vi "Process DAQ Data.vi"(0 "reset averaging":bool, 1 "Processing loop variables":T6 {"CurrInverter"."last updated" format="%<%H:%M\n%d/%m/%Y>T"; "CurrInverter"."set flag" items=["False", "True"]}, 2 "Data Rate 9775(S/s)":dbl=3.0 format="%#.6p", 3 "RawDAQData in":T16, 4 "Signal scaling":T15[](array[typedef]), 5 "error in":errorcluster, 6 "Data Rate 9215 (S/s)":dbl=1200000.0 format="%#.6p", 7 "ESR scaling":T14[](array[typedef]), 8 "Acquisition mode":T1, 11 "Use dummy Vout?":bool, 13 "Dummy Vrms":dbl=120.0) -> (10 "InverterWaveforms":T2, 15 "Processing loop vars out":T6 {"CurrInverter"."last updated" format="%<%H:%M\n%d/%m/%Y>T"; "CurrInverter"."set flag" items=["False", "True"]}, 16 "DataProcAuxData":T13[](array[typedef]), 18 "MeasData":T4, 19 "error out":errorcluster)   [LabVIEW 2019, in "Main.lvclass"]
doc: "Developed by Kevin Thompson\nkevin@thompsonengineering.net\n\nCopyright 2020\nThompson Engineering, LLC"
uses:
  Main.lvclass
  Common/DataTypes/RawDAQData--cluster.ctl
  Common/DataTypes/RawChannelData--cluster.ctl
  subvis/DataTypes/Gain control.ctl
  subvis/DataTypes/Processing loop variables--cluster.ctl
  subvis/DataTypes/averaging variables.ctl
  subvis/DataTypes/ESR alarm variables.ctl
  Common/DataTypes/Inverter database record v2--cluster.ctl
  Common/DataTypes/inverter info v2--cluster.ctl
  Common/DataTypes/inverter gain range--cluster.ctl
  Common/DataTypes/inverter offset range--cluster.ctl
  subvis/DataTypes/ESR scaling--cluster.ctl
  DataTypes/DataProcessAuxData--cluster.ctl
  Common/DataQ_SE/TD MeasData--cluster.ctl
  Common/DataTypes/InverterPhaseData--cluster.ctl
  Common/DataTypes/InverterWaveforms--cluster.ctl
  Common/DataTypes/ChannelWaveforms--cluster.ctl
  Common/DataTypes/Acquisition Mode--cluster.ctl
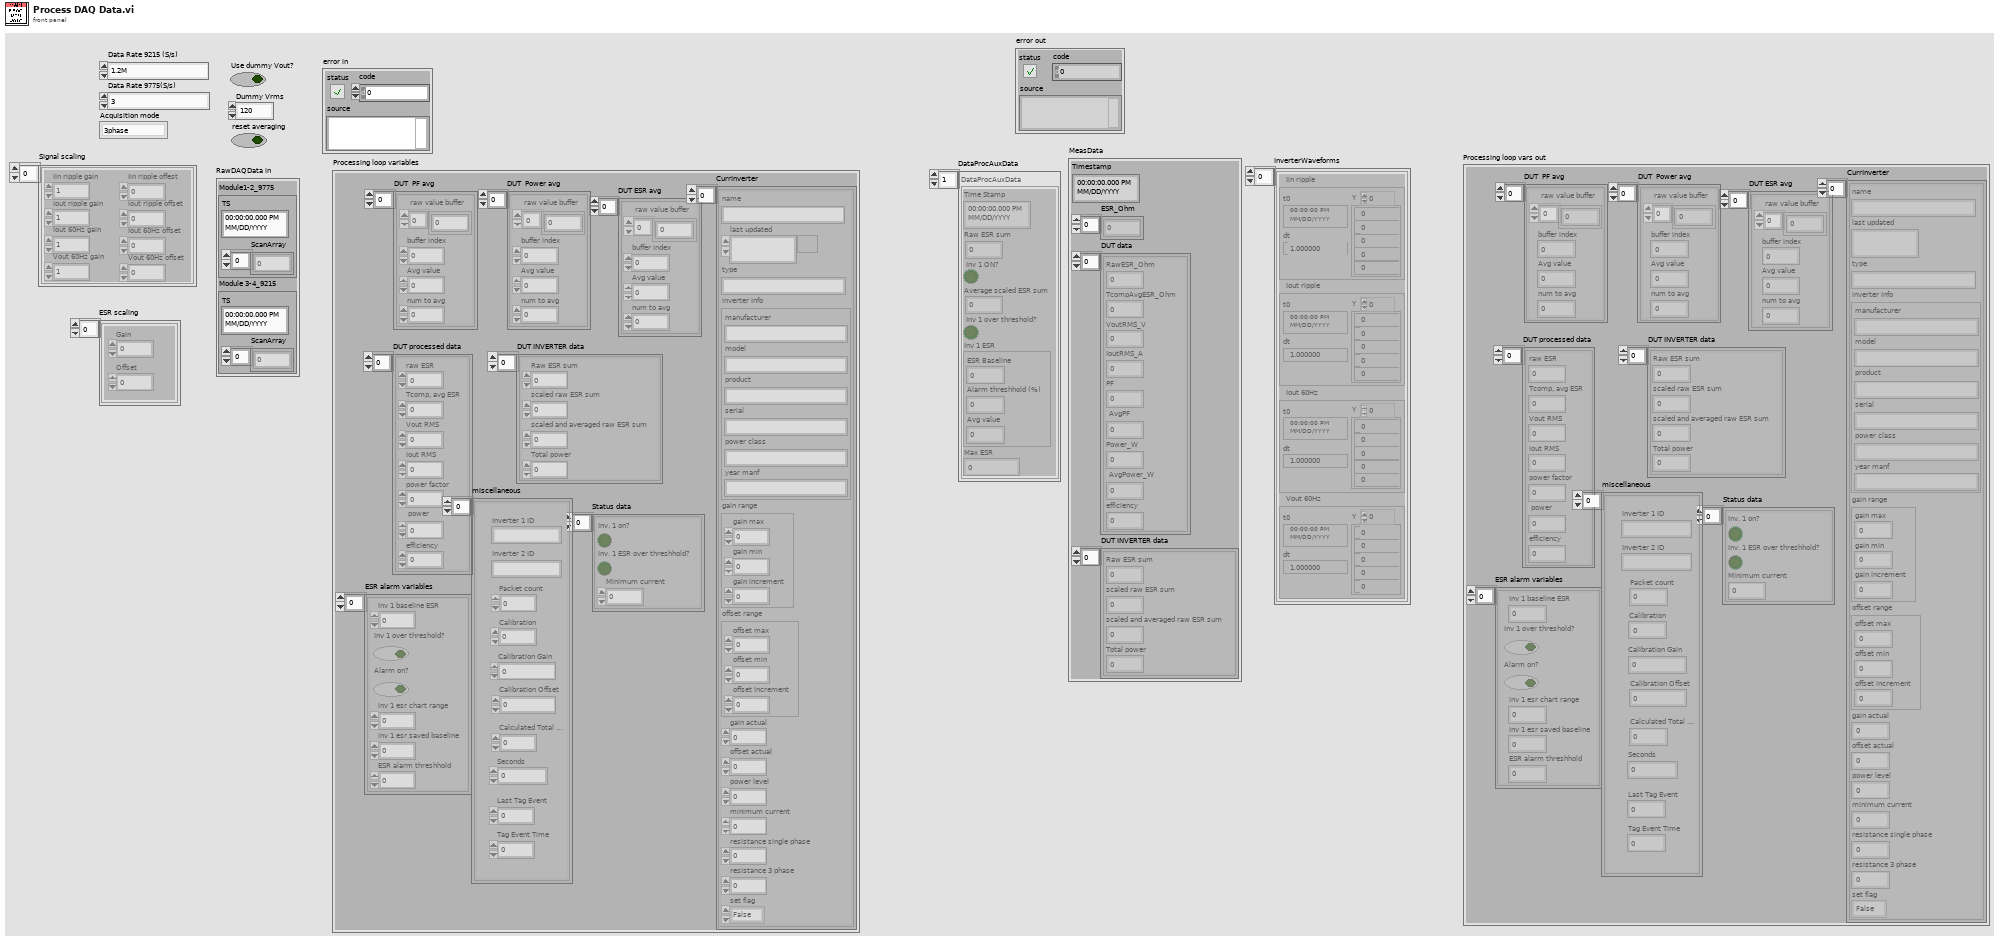
[diagram p1: front panel]
types:
  T1 = typedef "Acquisition Mode--cluster.ctl" = enum16{"3phase", "Single"}
  T2 = typedef "InverterWaveforms--cluster.ctl" = T3[]
  T3 = typedef "ChannelWaveforms--cluster.ctl" = cluster{"Iin ripple ":waveform(dbl), "Iout ripple ":waveform(dbl), "Iout 60Hz":waveform(dbl), "Vout 60Hz":waveform(dbl)}
  T4 = typedef "TD MeasData--cluster.ctl" = cluster{"Timestamp":timestamp, "ESR_Ohm":dbl[], "DUT data":T5[], "DUT INVERTER data":cluster{"Raw ESR sum":dbl, "scaled raw ESR sum":dbl, "scaled and averaged raw ESR sum":dbl, "Total power":dbl}[]}
  T5 = typedef "InverterPhaseData--cluster.ctl" = cluster{"RawESR_Ohm":dbl, "TcompAvgESR_Ohm":dbl, "VoutRMS_V":dbl, "IoutRMS_A":dbl, "PF":dbl, "AvgPF":dbl, "Power_W":dbl, "AvgPower_W":dbl, "efficiency":dbl}
  T6 = typedef "Main.lvclass/Processing loop variables--cluster.ctl" = cluster{"DUT ESR avg":T7[], "DUT  PF avg":T7[], "DUT  Power avg ":T7[], "DUT processed data":cluster{"raw ESR":dbl, "Tcomp, avg ESR":dbl, "Vout RMS":dbl, "Iout RMS":dbl, "power factor":dbl, "power":dbl, "efficiency":dbl}[], "ESR alarm variables":T8[], "Status data":cluster{"Inv. 1 on?":bool, "Inv. 1 ESR over threshhold?":bool, "Minimum current":dbl}[], "CurrInverter":T9[], "miscellaneous":cluster{"Inverter 1 ID":string, "Inverter 2 ID":string, "Packet count":u32, "Calibration":dbl, "Calibration Gain":dbl, "Calibration Offset":dbl, "Calculated Total Power":dbl, "Seconds":dbl, "Last Tag Event":dbl, "Tag Event Time":dbl}[], "DUT INVERTER data":cluster{"Raw ESR sum":dbl, "scaled raw ESR sum":dbl, "scaled and averaged raw ESR sum":dbl, "Total power":dbl}[]}
  T7 = typedef "Main.lvclass/averaging variables.ctl" = cluster{"raw value buffer":dbl[], "buffer index":i32, "Avg value":dbl, "num to avg":i32}
  T8 = typedef "Main.lvclass/ESR alarm variables.ctl" = cluster{"Inv 1 baseline ESR":dbl, "Inv 1 over threshold?":bool, "Alarm on?":bool, "inv 1 esr chart range":dbl, "inv 1 esr saved baseline":dbl, "ESR alarm threshhold":dbl}
  T9 = typedef "Inverter database record v2--cluster.ctl" = cluster{"name":string, "last updated":timestamp, "type":string, "inverter Info":T10, "gain range":T11, "offset range":T12, "gain actual":dbl, "offset actual":dbl, "power level":dbl, "minimum current":dbl, "resistance single phase":dbl, "resistance 3 phase":dbl, "set flag":u16}
  T10 = typedef "inverter info v2--cluster.ctl" = cluster{"manufacturer":string, "model":string, "product":string, "serial":string, "power class":string, "year manf":string}
  T11 = typedef "inverter gain range--cluster.ctl" = cluster{"gain max":dbl, "gain min":dbl, "gain increment":dbl}
  T12 = typedef "inverter offset range--cluster.ctl" = cluster{"offset max":dbl, "offset min":dbl, "offset increment":dbl}
  T13 = typedef "DataProcessAuxData--cluster.ctl" = cluster{"Time Stamp":timestamp, "Raw ESR sum":dbl, "Inv 1 ON?":bool, "Average scaled ESR sum":dbl, "Inv 1 over threshold?":bool, "Inv 1 ESR":cluster{"ESR Baseline":dbl, "Alarm threshhold (%)":dbl, "Avg value":dbl}, "Max ESR":dbl}
  T14 = typedef "Main.lvclass/ESR scaling--cluster.ctl" = cluster{"Gain":dbl, "Offset":dbl}
  T15 = typedef "Main.lvclass/Gain control.ctl" = cluster{"Iin ripple gain":dbl, "Iout ripple gain":dbl, "Iout 60Hz gain ":dbl, "Vout 60Hz gain ":dbl, "Iin ripple offest":dbl, "Iout ripple offset":dbl, "Iout 60Hz offset":dbl, "Vout 60Hz offset":dbl}
  T16 = typedef "RawDAQData--cluster.ctl" = cluster{"Module1-2_9775":T17, "Module 3-4_9215":T17}
  T17 = typedef "RawChannelData--cluster.ctl" = cluster{"TS":timestamp, "ScanArray":dbl[]}
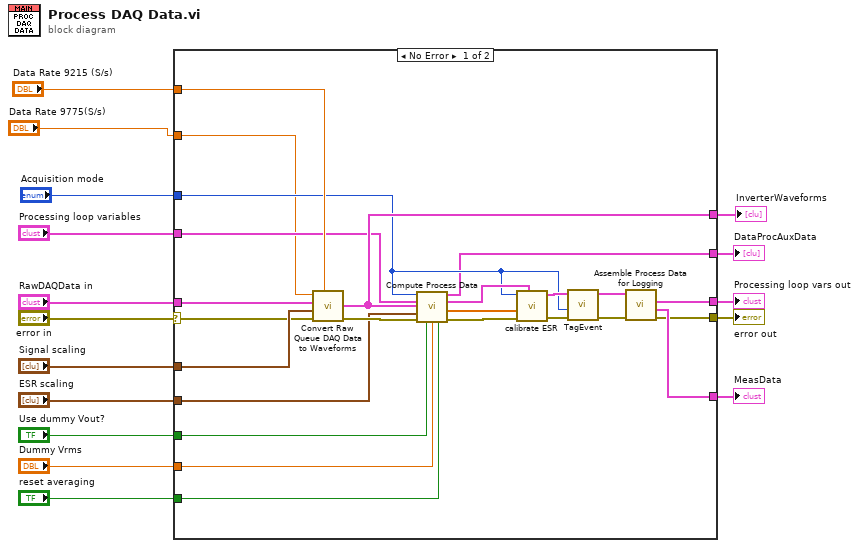
[diagram p0: block diagram]
diagram:
  n1 = case shown="No Error" "error in" {
    selector: "error in" -> [w28 w42]
    tunnel: "RawDAQData in" -> [w39 _]
    tunnel: "Data Rate 9215 (S/s)" -> [w38 _]
    tunnel: "Signal scaling" -> [w37 _]
    tunnel: "Processing loop variables" -> [w27 w41]
    tunnel: "ESR scaling" -> [w36 _]
    tunnel: "Use dummy Vout?" -> [w35 _]
    tunnel: "Dummy Vrms" -> [w34 _]
    tunnel: "reset averaging" -> [w33 _]
    tunnel: [w19 _] -> w8
    tunnel: [w32 w41] -> w7
    tunnel: [w31 _] -> w6
    tunnel: [w30 w42] -> w5
    tunnel: [w29 _] -> w4
    tunnel: "Acquisition mode" -> [w20 _]
    tunnel: "Data Rate 9775(S/s)" -> [w18 _]
    frame No Error {
      n2 = call "Convert Raw Queue DAQ Data to Waveforms.vi"("Data Rate 9215 (S/s)"=w38, "error in"=w28, "Signal scaling"=w37, "RawDAQData in"=w39, "Data Rate 9775(S/s)"=w18) -> ("error out"=w40:errorcluster, "InverterWaveforms out"=w29:T2)  [unwired: 5 in]
      n3 = call "Compute Process Data.vi"("Acquisition mode"=w20, "Processing loop variables"=w27, "InverterWaveforms"=w29, "ESR scaling"=w36, "error in (no error)"=w40, "Use dummy Vout?"=w35, "Dummy Vrms"=w34, "reset averaging"=w33) -> ("DataProcAuxData"=w19:T13[], "Processing loop vars out"=w25:T6, "Max ESR"=w17:dbl[], "error out"=w26:errorcluster)  [unwired: 4 in]
      n4 = call "calibrate ESR.vi"("Processing loop variables"=w25, "error in (no error)"=w26, "Max ESR"=w17, "Acquisition mode in"=w20) -> ("error out"=w24:errorcluster, "Processing loop vars out"=w23:T6)  [unwired: 6 in]
      n5 = call "TagEvent.vi"("error in"=w24, "Acquisition mode in"=w20, "Processing loop vars in"=w23) -> ("error out"=w21:errorcluster, "Processing loop vars out"=w22:T6)  [unwired: 7 in]
      n6 = call "Assemble Process Data for Logging.vi"("error in"=w21, "Processing loop variables"=w22) -> ("error out"=w30:errorcluster, "MeasData"=w31:T4, "Processing loop vars out"=w32:T6)  [unwired: 7 in]
    }
    frame Error {
    }
  }
  "error out" <- w5
  "DataProcAuxData" <- w8
  "Processing loop vars out" <- w7
  "MeasData" <- w6
  "InverterWaveforms" <- w4
